vi "Calculate_New_Positions.vi"(4 "C2":dbl, 6 "C1":dbl, 7 "Global best position":dbl, 8 "Inertial Coefficient":dbl, 9 "Best Particle Position":dbl[](array[numeric]), 10 "Current Particle Position":dbl[](array[numeric]), 11 "Current Particle Velocity":dbl[](array[numeric])) -> (2 "Updated Particle Positions":dbl[](array[numeric]), 3 "Updated Particle Velocities":dbl[](array[numeric]))   [LabVIEW 2011]
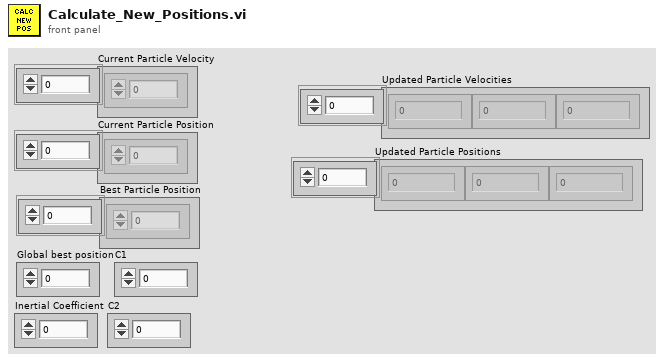
[diagram p1: front panel]
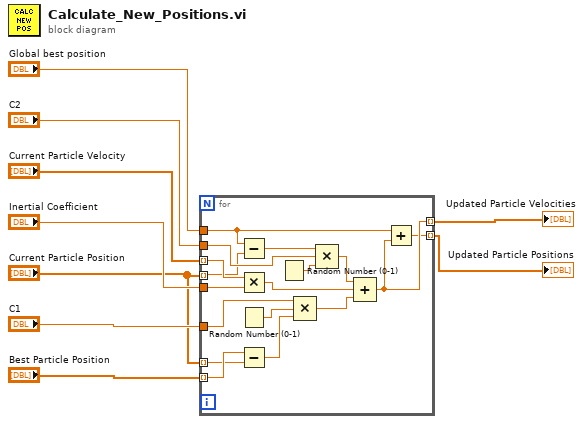
[diagram p0: block diagram]
diagram:
  n1 = for {
    tunnel: "Inertial Coefficient" -> [w26]
    tunnel: "Current Particle Velocity" -> [w25] mode=indexing
    tunnel: "C1" -> [w24]
    tunnel: "Best Particle Position" -> [w22] mode=indexing
    tunnel: "Current Particle Position" -> [w21] mode=indexing
    tunnel: "C2" -> [w16]
    tunnel: "Current Particle Position" -> [w14] mode=indexing
    tunnel: "Global best position" -> [w12]
    tunnel: [w11] -> w1 mode=indexing
    tunnel: [w10] -> w2 mode=indexing
    n2 = Subtract(x=w12, y=w14) -> (x-y=w15:dbl)
    n3 = Multiply(x=w25, y=w26) -> (x*y=w19:dbl)
    n4 = Random Number (0-1)() -> (number: 0 to 1=w23:dbl)
    n5 = Subtract(x=w22, y=w21) -> (x-y=w20:dbl)
    n6 = Random Number (0-1)() -> (number: 0 to 1=w17:dbl)
    n7 = Compound Arithmetic op=MULTIPLY(w24, w23, w20) -> (w18:dbl)
    n8 = Compound Arithmetic op=MULTIPLY(w15, w16, w17) -> (w13:dbl)
    n9 = Compound Arithmetic op=ADD(w13, w19, w18) -> (w11:dbl)
    n10 = Add(x=w12, y=w11) -> (x+y=w10:dbl)
  }
  "Updated Particle Positions" <- w2
  "Updated Particle Velocities" <- w1
